vi "nicrio_Mdk2Api_Command.vi"(0 "Write Data":u8, 2 "Comm Core I/O References":T2={"Command Interface"="Mod1/Command Interface", "Configuration Interface"="Mod1/Configuration Interface", "Debug Interface"="Mod1/Debug Interface", "Timing Interface"="Mod1/Timing Interface", "Status Interface"="Mod1/Status Interface", "DIO(7:0)"="Mod1/DIO(7:0)", "DIO0"="Mod1/DIO0", "DIO1"="Mod1/DIO1", "DIO2"="Mod1/DIO2", "DIO3"="Mod1/DIO3", "DIO4"="Mod1/DIO4", "DIO5"="Mod1/DIO5", "DIO6"="Mod1/DIO6", "DIO7"="Mod1/DIO7", "DIO8"="Mod1/DIO8"}, 5 "Command Type":T1 items=["Identify Module", "SPI Start", "SPI End", "SPI Wait", "SPI Byte", "SPI Byte & Start", "SPI Byte & End", "Change Mode", "Read EEPROM", "Write EEPROM"]) -> (4 "Read Data":u8)   [LabVIEW 2017]
uses:
  <vilib>/LabVIEW Targets/FPGA/cRIO/shared/nicrio_Mdk2Api/nicrio_Mdk2Api_IOReferences.ctl
  <vilib>/LabVIEW Targets/FPGA/cRIO/shared/nicrio_ModuleControls/nicrio_cRIO-Mdk2_CommandType.ctl
  <vilib>/rvi/eio/common/nirviEmuTemplateMethod_errors.vi
  <vilib>/eio/EIOMethodNode/EIOMethodNode.xnode
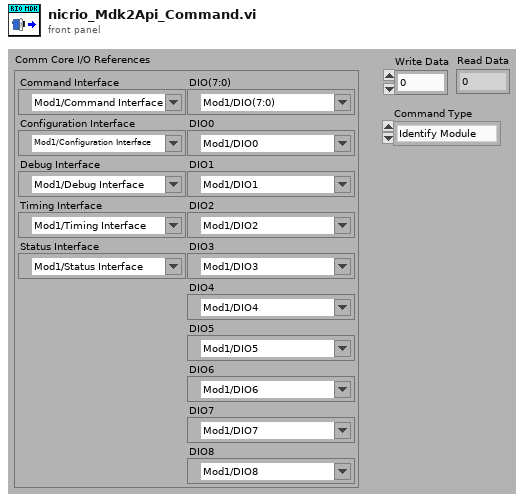
[diagram p1: front panel]
types:
  T1 = typedef "nicrio_cRIO-Mdk2_CommandType.ctl" = u8
  T2 = typedef "nicrio_Mdk2Api_IOReferences.ctl" = cluster{"Command Interface":refnum<k21>, "Configuration Interface":refnum<k21>, "Debug Interface":refnum<k21>, "Timing Interface":refnum<k21>, "Status Interface":refnum<k21>, "DIO(7:0)":refnum<k21>, "DIO0":refnum<k21>, "DIO1":refnum<k21>, "DIO2":refnum<k21>, "DIO3":refnum<k21>, "DIO4":refnum<k21>, "DIO5":refnum<k21>, "DIO6":refnum<k21>, "DIO7":refnum<k21>, "DIO8":refnum<k21>}
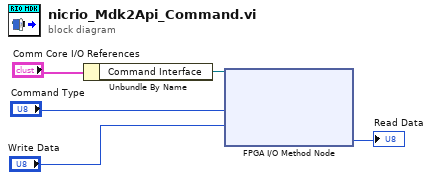
[diagram p0: block diagram]
diagram:
  n1 = Unbundle By Name("Comm Core I/O References") -> ("Command Interface"=w4:refnum<k21>)
  n2 = xnode "FPGA I/O Method Node"("FPGA I/O In"=w4, "Command Type"="Command Type", "Write Data"="Write Data") -> ("Read Data"=→"Read Data":u8)  [unwired: 1 out]
